vi "powermeter.vi"() -> ()   [LabVIEW 2015]
uses:
  <vilib>/Platform/TimedLoop/XDataNode/timing_clust.ctl
  <vilib>/Platform/TimedLoop/XDataNode/nitl_modes.ctl
  <vilib>/Platform/TimedLoop/XDataNode/wakeup.ctl
  <vilib>/Utility/file.llb/Write To Spreadsheet File (string).vi
  <vilib>/Utility/file.llb/Write To Spreadsheet File (DBL).vi
  <vilib>/platform/TimedLoop/XDataNode/XDataNode.xnode
  <vilib>/Platform/TimedLoop/XDataNode/XDNodeRunTimeDep.lvlib
panel:
  out "Wavelength (nm):":dbl caption="Wavelength"
  out "Beam Diameter (sq mm):":dbl caption="Beam Diameter"
  out "Frequency:":dbl caption="Frequency"
  out "Power:":dbl caption="Power"
  in  "stop":bool
  in  "About Button":bool
  in  "Save Button":bool
  in  "ClearData":bool
  in  "Take Data":bool
  in  "Wavelength (nm):":dbl caption="Wavelength (0.0)"
  in  "Power to Measure (W):":dbl=1e-09 caption="Power to Measure (0.0)" min=1e-09 max=0.1 step=0.1
  in  "SetPowerRange":bool
  in  "SetWavelength":bool
  out "Waveform Graph":dbl[](graph)
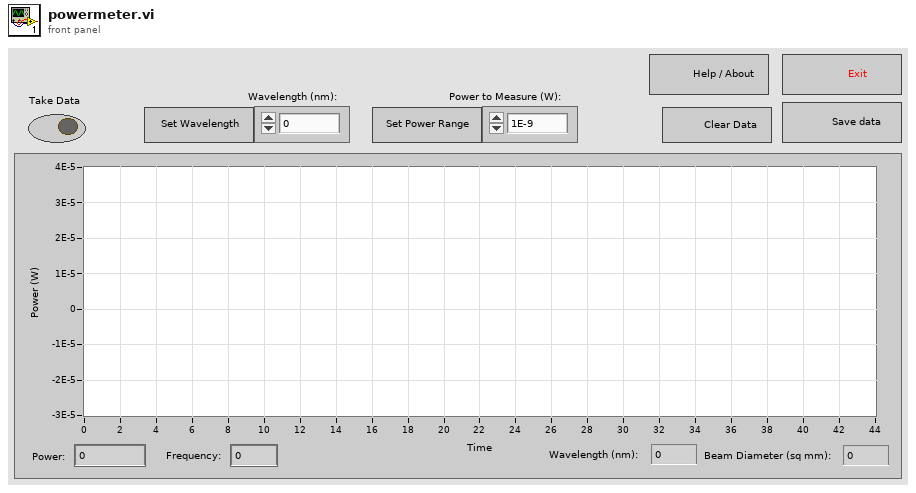
[diagram p1: front panel]
types:
  T1 = typedef "XDNodeRunTimeDep.lvlib/timing_clust.ctl" = cluster{"Expected End [f-1]":u64, "Actual End [f-1]":u64, "Finished Late? [f-1]":bool, "Expected End [i-1]":u64, "Actual End [i-1]":u64, "Finished Late? [i-1]":bool, "Expected Start [i]":u64, "Actual Start [i]":u64, "Expected Start [f]":u64, "Actual Start [f]":u64, "Source Name":string, "Structure Name":string, "Period":i64, "Deadline":i64, "Offset":i64, "Start":i64, "Priority":i32, "Timeout":i32, "Mode":T2, "Wakeup Reason":T3, "Error":errorcluster, "Source Type":string, "Secondary Source Type":string, "Global End Time":u64, "Global Start Time":u64, "Frame Duration":u64, "Iteration Duration":u64, "Assigned CPU":i32, "I/O Scan Engine Mode":u32}
  T2 = typedef "XDNodeRunTimeDep.lvlib/nitl_modes.ctl" = enum32{"No Change", "Process missed periods, maintain original phase", "Discard missed periods, maintain original phase", "Process missed periods, ignore original phase", "Discard missed periods, ignore original phase"}
  T3 = typedef "XDNodeRunTimeDep.lvlib/wakeup.ctl" = enum32{"Normal", "Aborted", "Asynchronous wakeup", "Timing source error", "Timed loop error", "Timeout"}
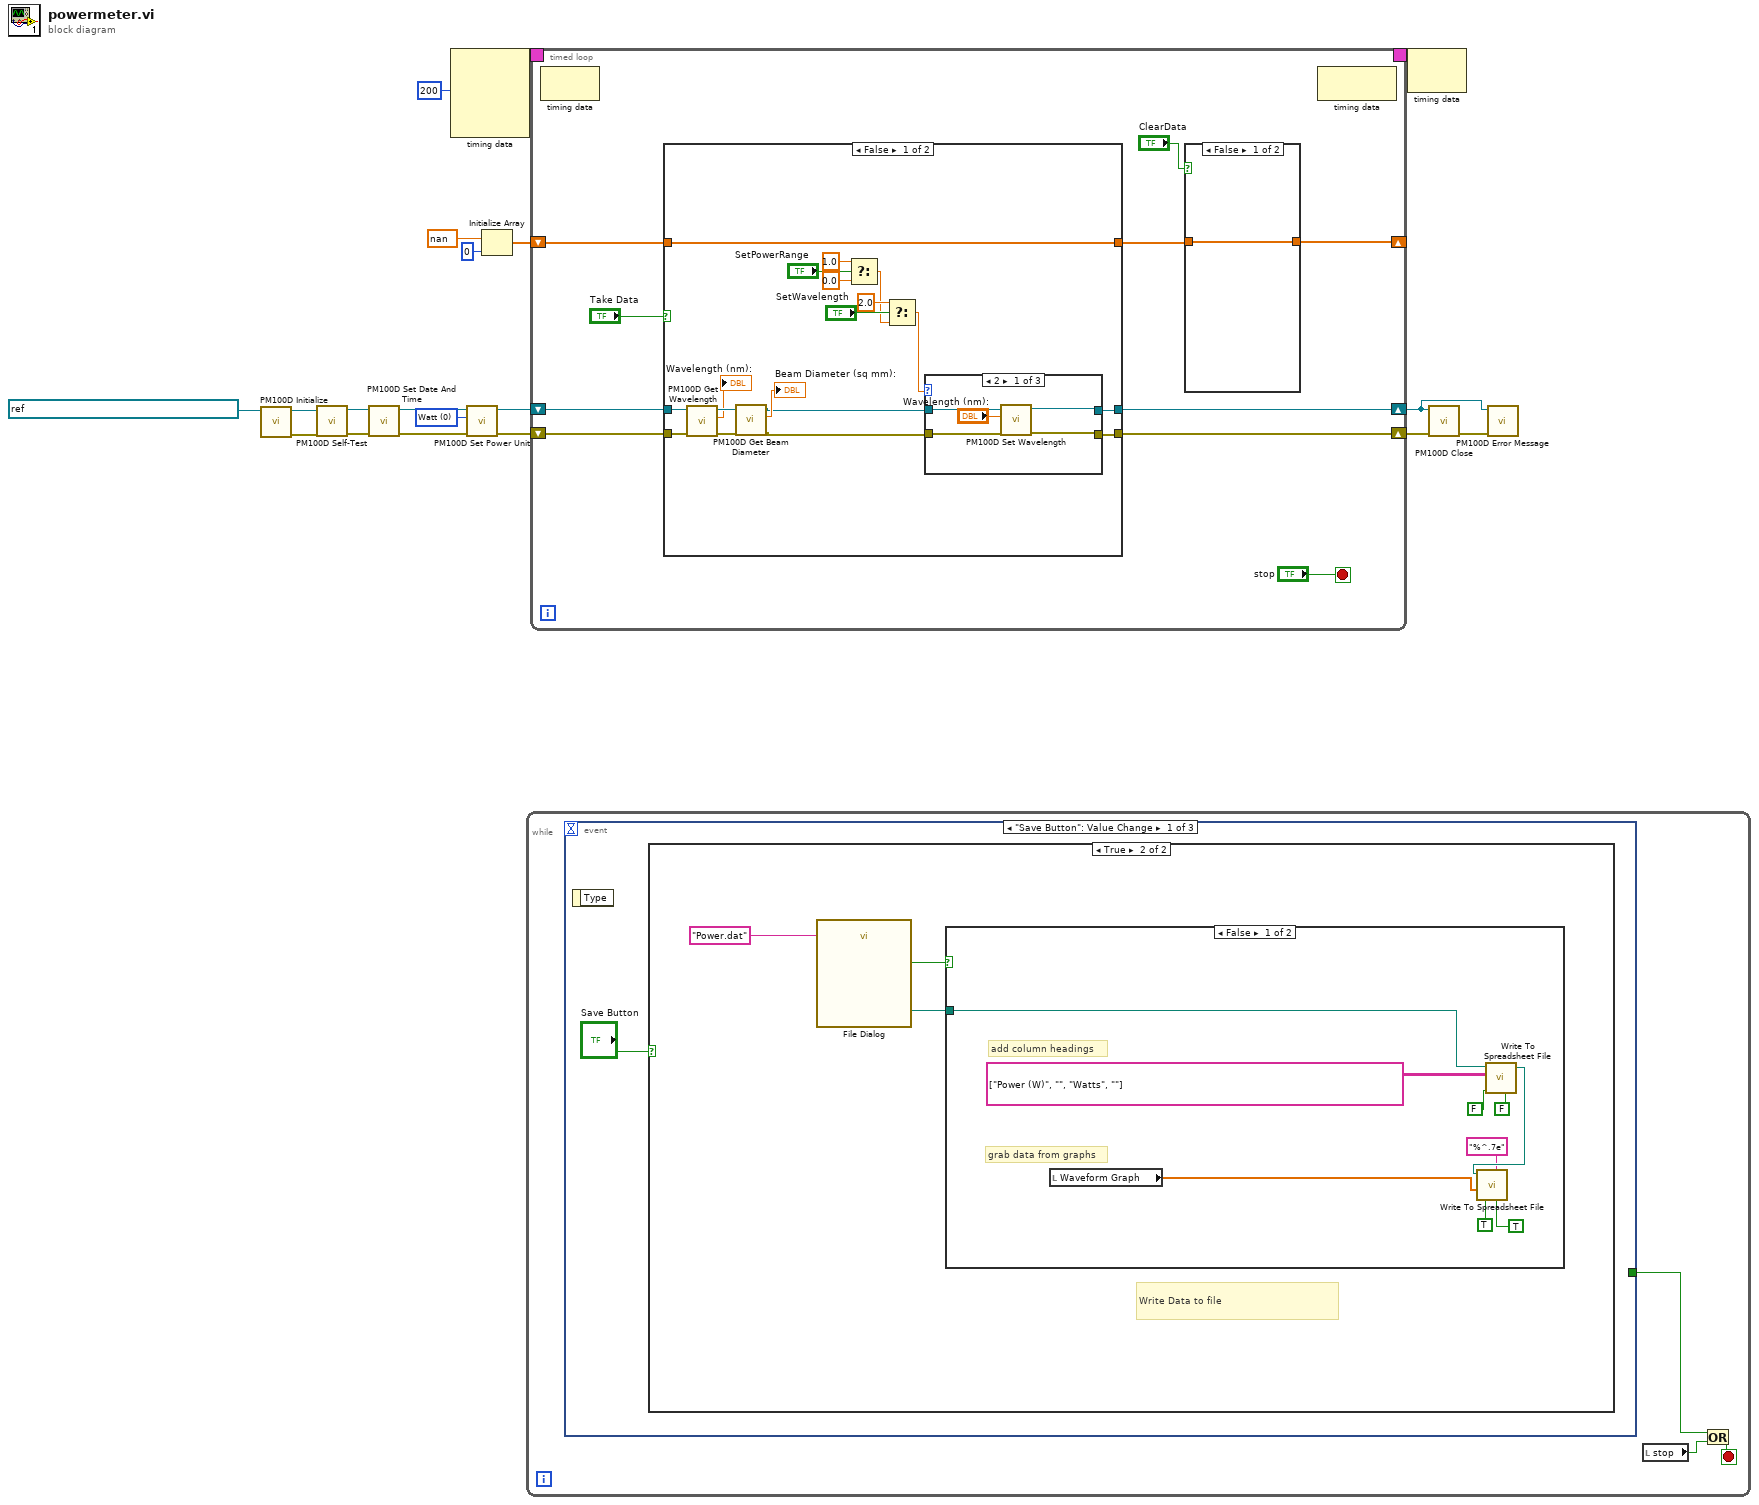
[diagram p0: block diagram]
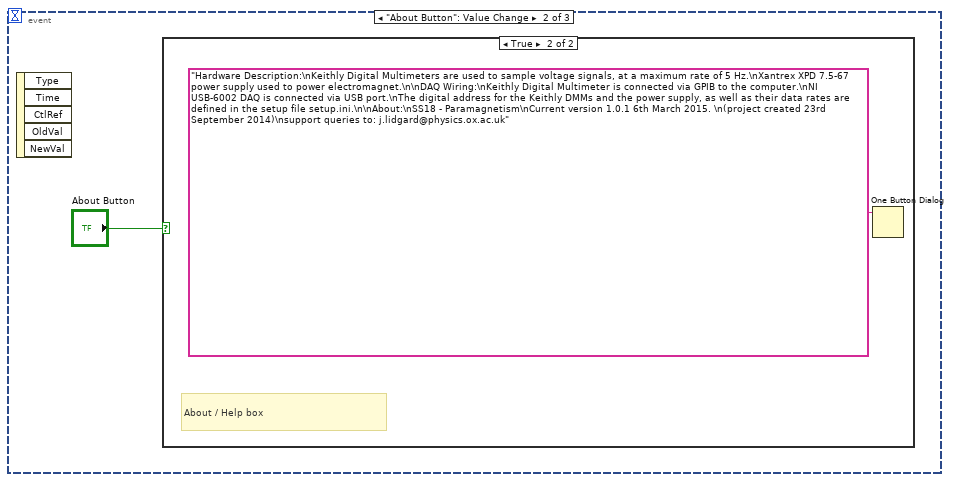
[diagram p4: hidden frame]
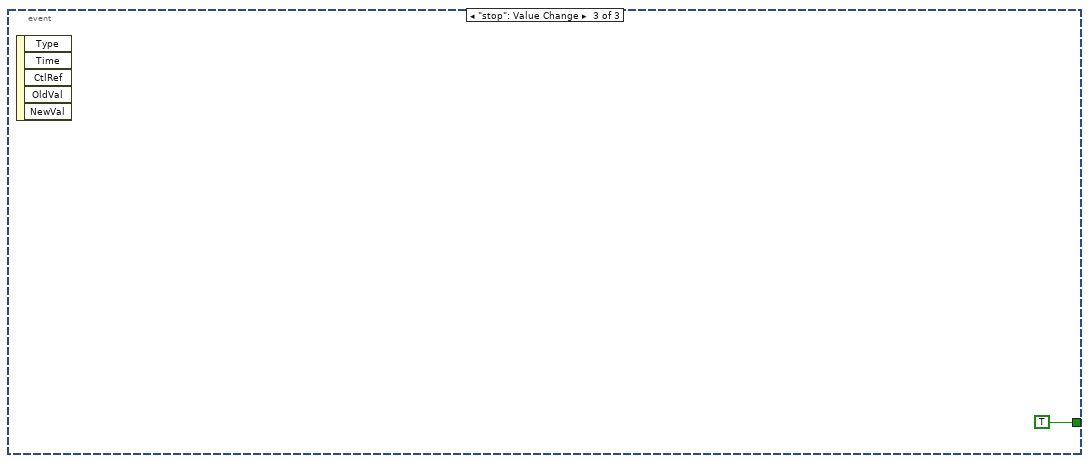
[diagram p6: hidden frame]
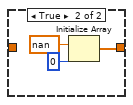
[diagram p7: hidden frame]
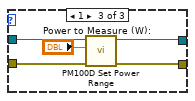
[diagram p9: hidden frame]
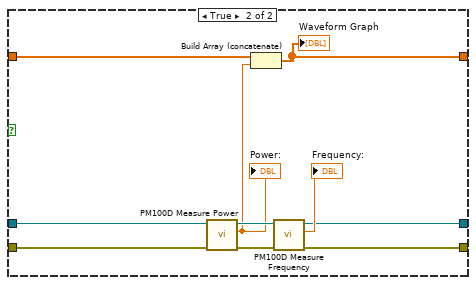
[diagram p10: hidden frame]
diagram:
  w1 = i16 0 items=["Watt", "dBm"] ("Power Unit (Watt)")
  n1 = call "PM100D Initialize.vi"("resource name"=refnum<visa-resource-name> "USB0::0x1313::0x8078::P0005368::INSTR") -> ("error out"=w17:errorcluster, "instrument handle out"=w19:refnum<visa-resource-name>)  [unwired: 9 in]
  n2 = call "PM100D Self-Test.vi"("error in (no error)"=w17, "instrument handle"=w19) -> ("error out"=w16:errorcluster, "instrument handle out"=w18:refnum<visa-resource-name>)  [unwired: 6 in, 2 out]
  n3 = call "PM100D Set Date And Time.vi"("error in (no error)"=w16, "instrument handle"=w18) -> ("error out"=w3:errorcluster, "instrument handle out"=w5:refnum<visa-resource-name>)  [unwired: 8 in]
  n4 = node-c288(i64 200 ("Period")) -> (w11:T1)  [unwired: 3 in]
  n5 = call "PM100D Set Power Unit.vi"("error in (no error)"=w3, "Power Unit (Watt)"=w1, "instrument handle"=w5) -> ("error out"=w2:errorcluster, "instrument handle out"=w4:refnum<visa-resource-name>)  [unwired: 7 in]
  n6 = Initialize Array(nan ("element"), 0 ("dimension size")) -> (w8:dbl[])
  n7 = while {
    stop <- w21 stop-if-true
    n8 = event shown="[0] \"Save Button\": Value Change" {
      selector: _ -> [_ _ _]
      dyn-events: _ -> [_ _ _]
      timeout: _ -> [_ _ _]
      tunnel: [_ _ TRUE ("x")] -> w20
      event "Save Button": Value Change {
        n9 = event-data() -> ()  [unwired: 1 in, 1 out]
        n10 = case shown="True" "Save Button" {
          frame False {
          }
          frame True {
            # "Write Data to file"
            n11 = call "File Dialog"("default name"="Power.dat") -> ("selected path"=w26:path, "cancelled"=w24:bool)  [unwired: 11 in, 2 out]
            n12 = case shown="False" w24 {
              tunnel: w26 -> [w28 _]
              frame False {
                # "add column headings"
                # "grab data from graphs"
                n13 = local read "Waveform Graph"() -> (w27:dbl[])
                n14 = call-poly <vilib>:"Write To Spreadsheet File.vi"("transpose? (no:F)"=FALSE, "append to file? (new file:F)"=FALSE, "2D data"=string[][] [["Power (W)", ""], ["Watts", ""]], "file path (dialog if empty)"=w28) -> ("new file path (Not A Path if cancelled)"=w35:path)  [unwired: 4 in]
                n15 = call-poly <vilib>:"Write To Spreadsheet File.vi"("transpose? (no:F)"=TRUE, "format (%.3f)"="%^.7e", "append to file? (new file:F)"=TRUE, "1D data"=w27, "file path (dialog if empty)"=w35) -> ()  [unwired: 3 in, 1 out]
              }
              frame True {
              }
            }
          }
        }
      }
      event "About Button": Value Change {
        n16 = event-data() -> ()  [unwired: 1 in, 5 out]
        n17 = case shown="True" "About Button" {
          frame False {
          }
          frame True {
            # "About / Help box"
            n18 = One Button Dialog(message="Hardware Description:\nKeithly Digital Multimeters are used to sample voltage signals, at a maximum rate of 5 Hz.\nXantrex XPD 7.5-67 power supply used to power electromagnet.\n\nDAQ Wiring:\nKeithly Digital Multimeter is connected via GPIB to the computer.\nNI USB-6002 DAQ is connected via USB port.\nThe digital address for the Keithly DMMs and the power supply, as well as their data rates are defined in the setup file setup.ini.\n\nAbout:\nSS18 - Paramagnetism\nCurrent version 1.0.1 6th March 2015. \n(project created 23rd September 2014)\nsupport queries to: j.lidgard@physics.ox.ac.uk" ("format string")) -> ()  [unwired: 1 in, 1 out]
          }
        }
      }
      event "stop": Value Change {
        n19 = event-data() -> ()  [unwired: 1 in, 5 out]
      }
    }
    n20 = local read "stop"() -> (w22:bool)
    n21 = Or(x=w20, y=w22) -> (x .or. y?=w21:bool)
  }
  n22 = timed-loop {
    shift-right: [w45] -> w13
    shift-left: w4 -> [w48]
    shift-right: [w44] -> w15
    shift-left: w2 -> [w47]
    timing: w11 -> [_]
    timing-out: [_] -> w10
    shift-right: [w40] -> _
    shift-left: w8 -> [w46]
    stop <- "stop" stop-if-true
    n23 = node-c288() -> ()  [unwired: 1 in, 1 out]
    n24 = case shown="False" "Take Data" {
      tunnel: [w70 w86] -> w45
      tunnel: [w69 w85] -> w44
      tunnel: w48 -> [w60 w84]
      tunnel: w47 -> [w58 w83]
      tunnel: w46 -> [w61 w92]
      tunnel: [w61 w87] -> w41
      frame False {
        n25 = call "PM100D Get Wavelength.vi"("error in (no error)"=w58, "instrument handle"=w60) -> ("error out"=w57:errorcluster, "Wavelength"=→"Wavelength (nm):":dbl, "instrument handle out"=w59:refnum<visa-resource-name>)  [unwired: 7 in]
        n26 = call "PM100D Get Beam Diameter.vi"("error in (no error)"=w57, "instrument handle"=w59) -> ("error out"=w53:errorcluster, "Beam Diameter"=→"Beam Diameter (sq mm):":dbl, "instrument handle out"=w54:refnum<visa-resource-name>)  [unwired: 7 in]
        n27 = Select(t=1.0, s="SetPowerRange", f=0.0) -> (s? t:f=w63:dbl)
        n28 = Select(t=2.0, s="SetWavelength", f=w63) -> (s? t:f=w62:dbl)
        n29 = case shown="2" w62 {
          tunnel: w54 -> [w75 w77 w82]
          tunnel: [w72 w77 w79] -> w70
          tunnel: w53 -> [w74 w76 w81]
          tunnel: [w73 w76 w80] -> w69
          frame 2 {
            n30 = call "PM100D Set Wavelength.vi"("error in (no error)"=w74, "Wavelength (0.0)"="Wavelength (nm):", "instrument handle"=w75) -> ("error out"=w73:errorcluster, "instrument handle out"=w72:refnum<visa-resource-name>)  [unwired: 7 in]
          }
          frame 0, Default {
          }
          frame 1 {
            n31 = call "PM100D Set Power Range.vi"("error in (no error)"=w81, "Power to Measure (0.0)"="Power to Measure (W):", "instrument handle"=w82) -> ("error out"=w80:errorcluster, "instrument handle out"=w79:refnum<visa-resource-name>)  [unwired: 7 in]
          }
        }
      }
      frame True {
        n32 = call "PM100D Measure Power.vi"("error in (no error)"=w83, "instrument handle"=w84) -> ("error out"=w89:errorcluster, "Power"=w88:dbl, "instrument handle out"=w90:refnum<visa-resource-name>)  [unwired: 7 in]
        "Power:" <- w88
        n33 = Build Array (concatenate)(w92, w88) -> (w87:dbl[])
        "Waveform Graph" <- w87
        n34 = call "PM100D Measure Frequency.vi"("error in (no error)"=w89, "instrument handle"=w90) -> ("error out"=w85:errorcluster, "Frequency"=→"Frequency:":dbl, "instrument handle out"=w86:refnum<visa-resource-name>)  [unwired: 7 in]
      }
    }
    n35 = case shown="False" "ClearData" {
      tunnel: w41 -> [w49 _]
      tunnel: [w49 w52] -> w40
      frame False {
      }
      frame True {
        n36 = Initialize Array(nan ("element"), 0 ("dimension size")) -> (w52:dbl[])
      }
    }
    n37 = node-c288() -> ()  [unwired: 1 in, 1 out]
  }
  n38 = node-c288(w10) -> ()  [unwired: 1 out]
  n39 = call "PM100D Close.vi"("error in (no error)"=w15, "instrument handle"=w13) -> ("error out"=w14:errorcluster)  [unwired: 9 in]
  n40 = call "PM100D Error Message.vi"("error in (no error)"=w14, "instrument handle"=w13) -> ()  [unwired: 7 in, 3 out]
